vi "Movimiento_Heliptica.vi"() -> ()   [LabVIEW 2021]
panel:
  in  "Numeric 2":dbl
  in  "Numeric":dbl
  in  "stop":bool
  out "Boolean":bool
  # "MENDOZA MEZA MANUEL EVERARDO"
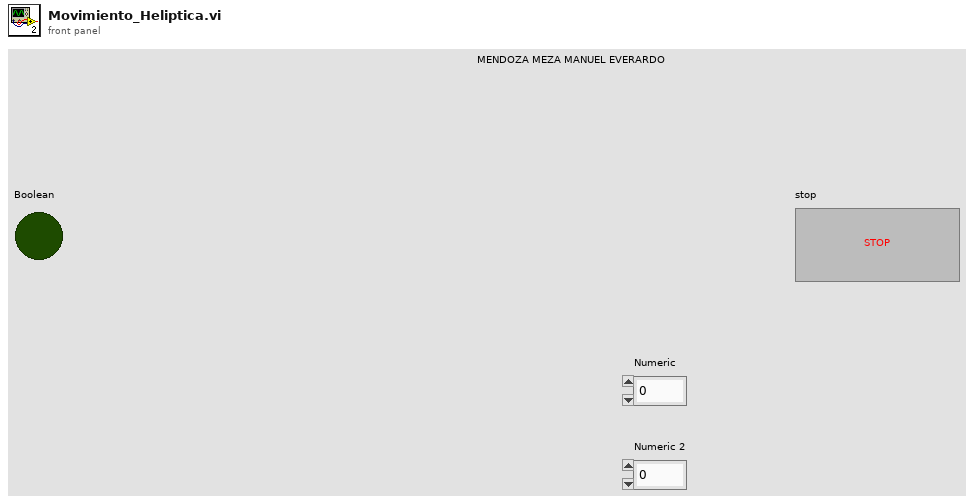
[diagram p1: front panel]
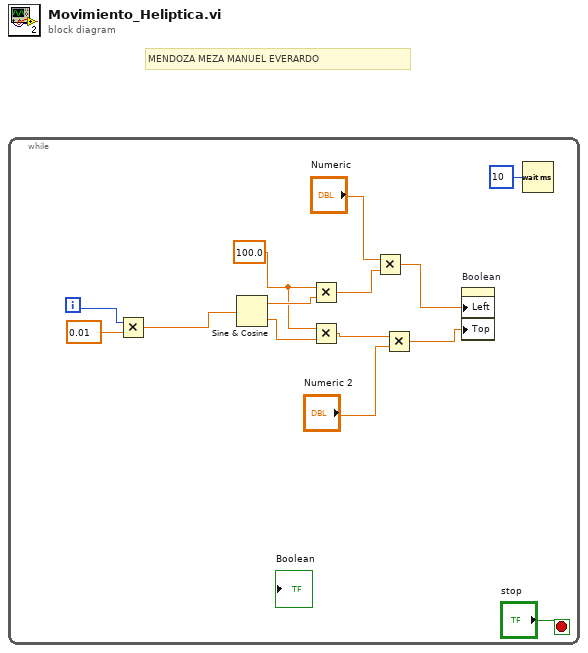
[diagram p0: block diagram]
diagram:
  # "MENDOZA MEZA MANUEL EVERARDO"
  n1 = while {
    i -> [w8]
    stop <- "stop" stop-if-true
    w10 = 100.0 ("y")
    n2 = Multiply(x=w8, y=0.01) -> (x*y=w7:dbl)
    n3 = Sine & Cosine(0:w7) -> (1:w11:dbl, 2:w9:dbl)
    n4 = Multiply(x=w10, y=w11) -> (x*y=w6:dbl)
    n5 = Multiply(x=w10, y=w9) -> (x*y=w2:dbl)
    n6 = Multiply(x="Numeric", y=w6) -> (x*y=w4:dbl)
    n7 = Multiply(x=w2, y="Numeric 2") -> (x*y=w3:dbl)
    n8 = property on="Boolean" class="Bool (strict)"("Left"=w4, "Top"=w3) -> ()  [unwired: 2 in, 2 out]
    n9 = Wait (ms)(milliseconds to wait=u32 10) -> ()  [unwired: 1 out]
  }
